vi "uTTA_Calibration.vi"() -> ()   [LabVIEW 2021]
uses:
  <vilib>/Utility/miscctls.llb/LVPointTypeDef.ctl
  uTTA_Device_Driver/CTL_uTTA_OperatingMode.ctl
  <vilib>/Analysis/6fits.llb/Curve Fitting Criteria.ctl
  <vilib>/Analysis/NI_AALBase.lvlib
  <vilib>/Analysis/NI_AALPro.lvlib
panel:
  out "Trys":i32
  out "PGA":i32
  out "Measurement Active":bool
  out "Queue":i32
  out "Communication Error":errorcluster
  out "RunTime Error":errorcluster
  out "Last Message":string
  in  "Tab Control":T1(tab)
  in  "uTTA COM":refnum<visa-resource-name>
  in  "VISA Function Gen":refnum<visa-resource-name>
  in  "Storage_Path":path=path "C:/temp/Octave_Thermal_Modelling/Measurement_Data"
  in  "VISA DMM":refnum<visa-resource-name>
  in  "Cal Adapter":bool
  in  "DAC Increments":dbl=0.025 caption="DAC Voltage\nIncrement" min=0.001 max=1.0 format="%.3p V/Step"
  in  "Start ADC Cal":bool
  out "Calibration of Channel":u32
  out "PGA setting":u32
  out "ADC Cal.":cluster{"Voltage mean":dbl, "mean":dbl}(graph)
  out "Ref. Voltage":dbl format="%#_6pV"
  out "ADC slope":dbl format="%#_4pV/Digit"
  out "ADC lin. res":dbl caption="ADC linearization\nresidue" format="%.3p"
  out "ADC intercept":dbl format="%#_6pV"
  out "PGA":u32
  out "ADC_Variance":dbl[](array[numeric]) format="%#.2g"
  out "Temp_Variance":dbl[](array[numeric]) format="%#.2g°C"
  out "Temp_Values":dbl[](array[numeric]) format="%#.1g°C"
  out "ADC_Values":dbl[](array[numeric]) format="%#.2g"
  out "Channel":u32
  in  "Complete Cal":bool
  out "Total Measurements":u32
  in  "Shunt Resistance":dbl format="%#_3pOhm"
  in  "Get Measurement":bool
  out "ADC Cal. 2":cluster{"Voltage mean":dbl, "mean":dbl}(graph)
  out "ADC_Values 2":dbl[](array[numeric]) format="%#.2g"
  out "ADC_Variance 2":dbl[](array[numeric]) format="%#.2g"
  in  "Start":bool
  out "Status":string="Exit"
  in  "stop":bool
  # "1. Connect the function generator with a 50Ohm Terminator and a BNC Y-Adaptor to the input of the uTTA.\n2. Connect a ground lead to the outer Conductor of the BNC line to provide propper grounding\n3. Start the calibration"
  # "1. Connect a power supply through a low resistance value shunt ( 10-100mOhm) to the JUT Current Input (J107) of uTTA.\n2. Connect the ground of the power supply to J106 of uTTA.\n3. Connect the sense leads of your multimeter to the sense terminals of the shunt.\n4. Set the power supply to a low current setting (~100mA).\n5. Get a measurement\n6. Set a higher current to the power supply. Steps of 1A to 2A should be sufficient.\n7. Repeat steps 5 and 6 multiple times until you have a good number of measurements.\n8. To finalize the calibration press \"Complete Calibration\"."
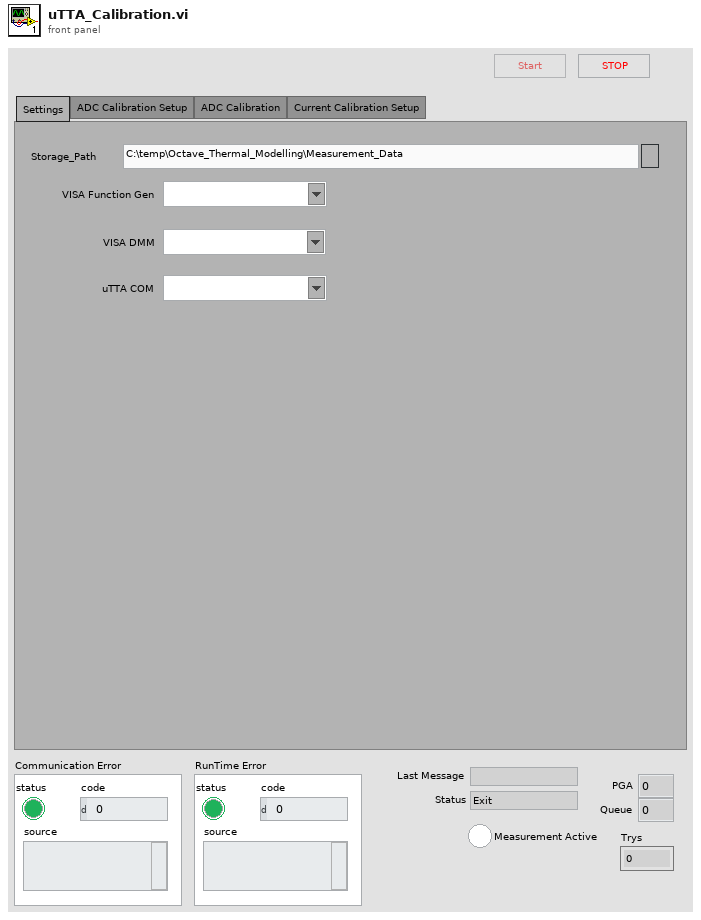
[diagram p1: front panel]
types:
  T1 = enum32{"Settings", "ADC Calibration Setup", "ADC Calibration", "Current Calibration Setup"}
  T2 = typedef "LVPointTypeDef.ctl" = cluster{"Horizontal":i16, "Vertical":i16}
  T3 = cluster{"ADC Values":i16[][], "Temperatures":dbl[][]}
  T4 = typedef "CTL_uTTA_OperatingMode.ctl" = enum16{"NORMAL", "CALIBRATION"}
  T5 = enum8{"Enabled", "Disabled", "Disabled and Grayed Out"}
  T6 = enum16{"open", "open or create", "create or replace", "create", "open (read-only)"}
  T7 = typedef "NI_AALPro.lvlib/Curve Fitting Criteria.ctl" = u16
  T8 = cluster{"CH0  CURRENT":i16[], "CH1 VOLTAGE":i16[]}
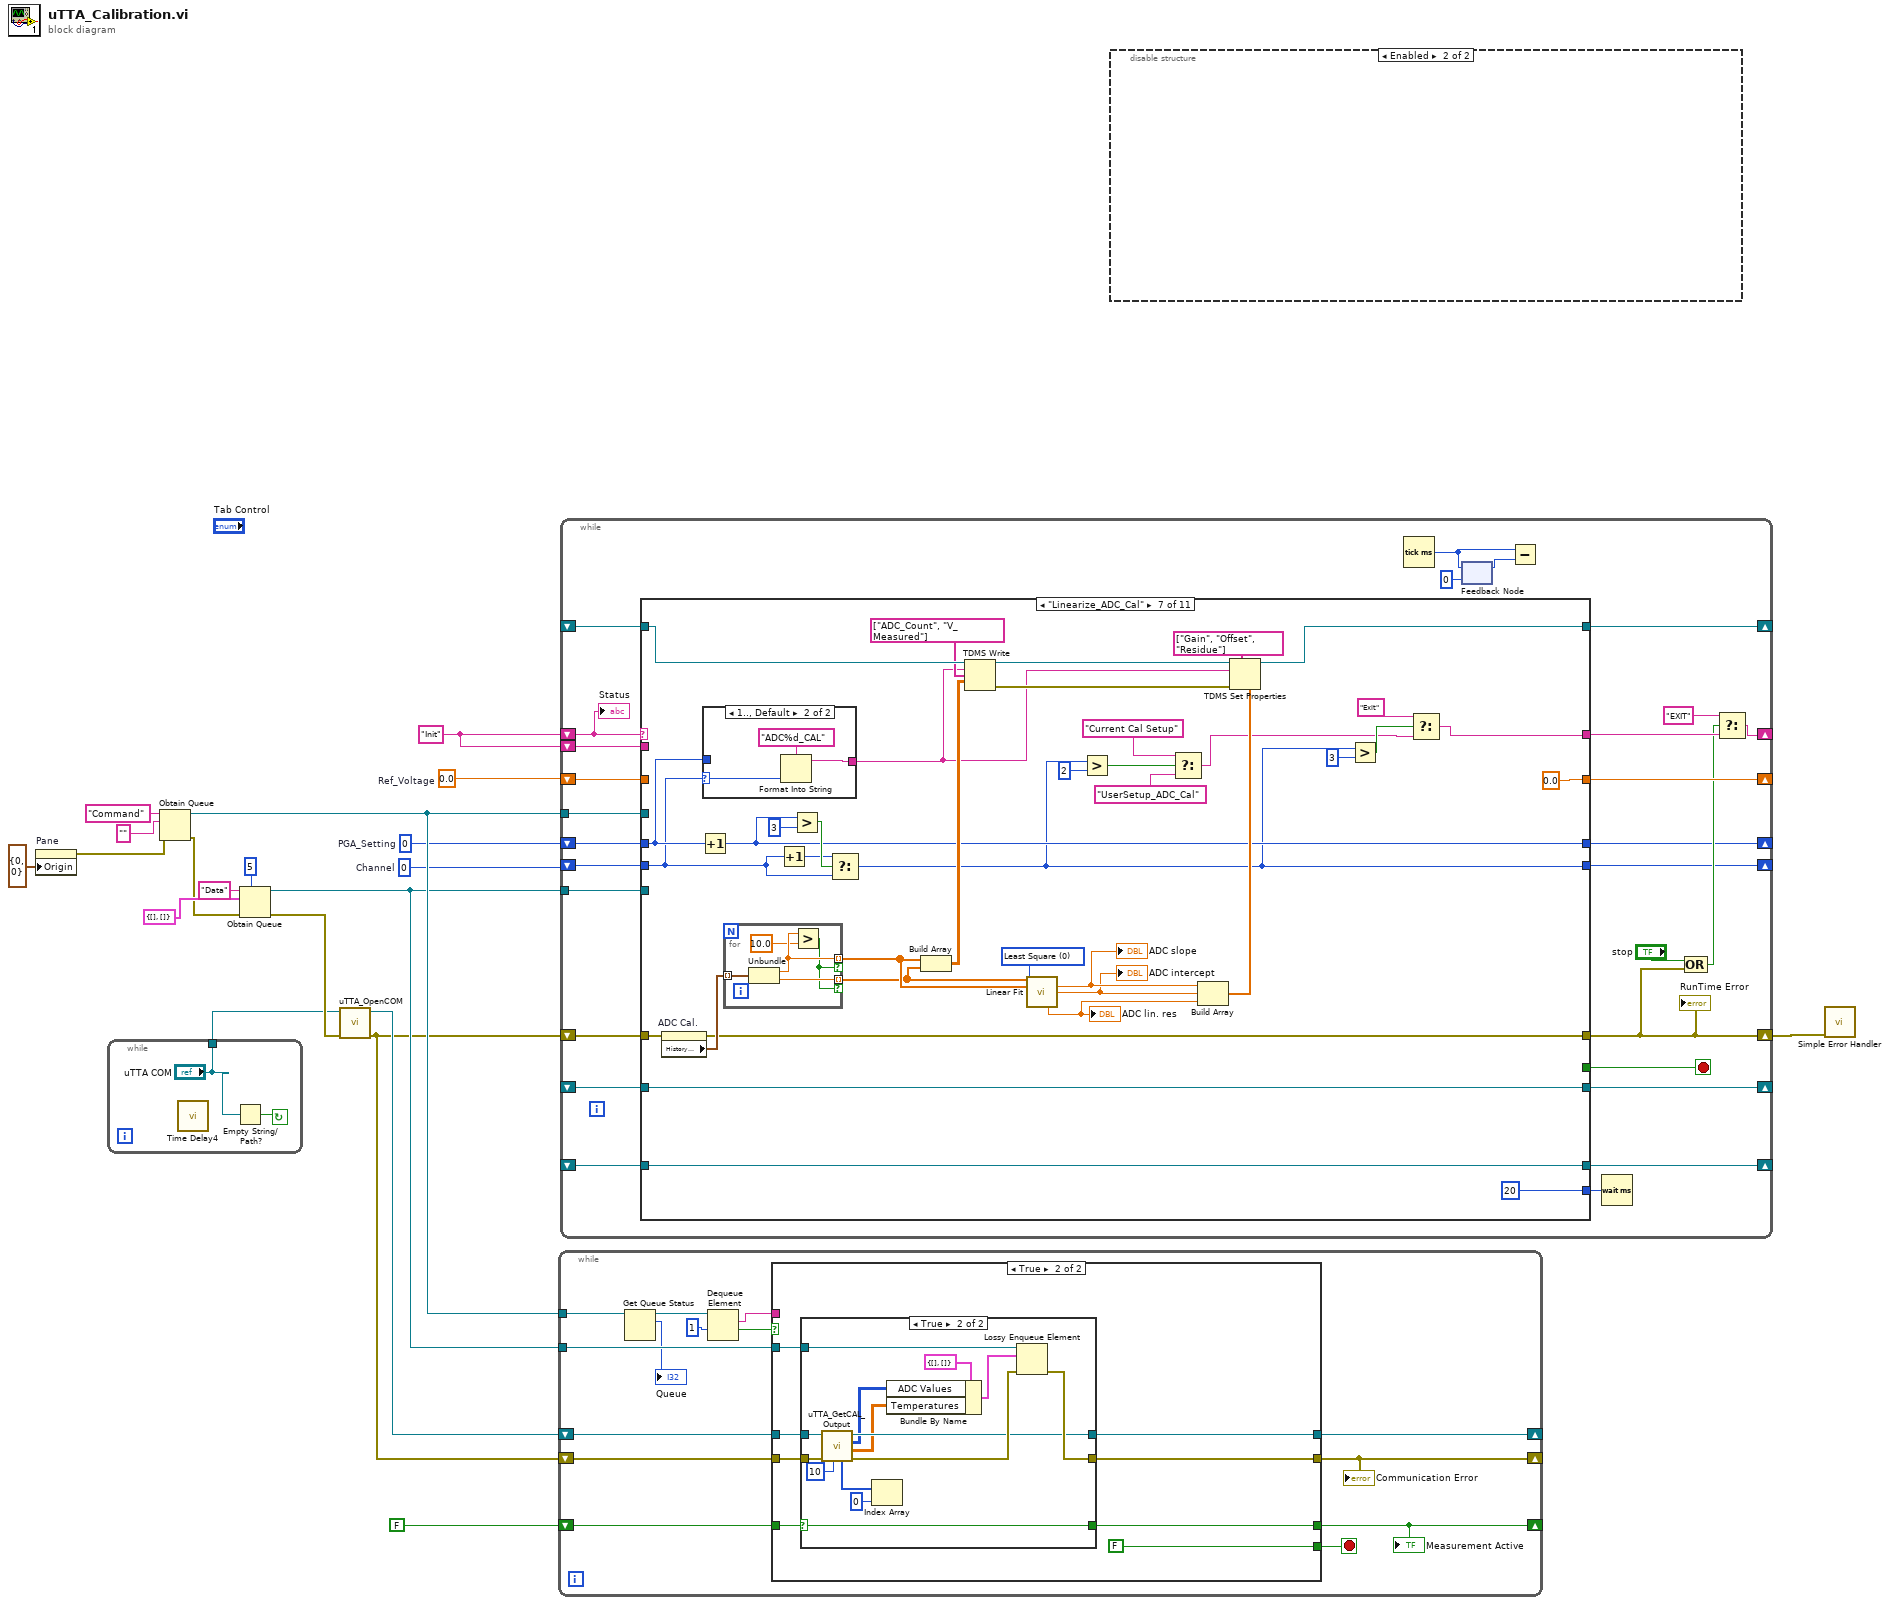
[diagram p0: block diagram]
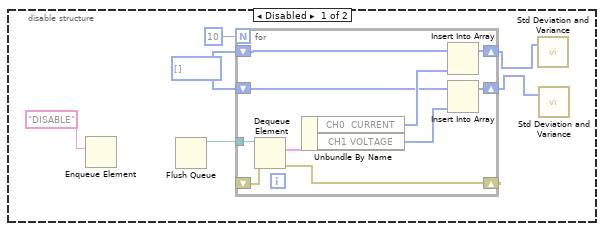
[diagram p2: hidden frame]
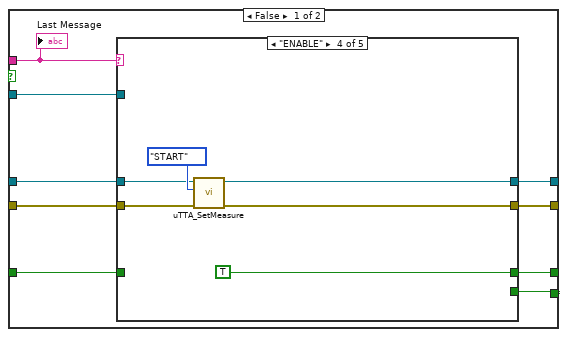
[diagram p3: hidden frame]
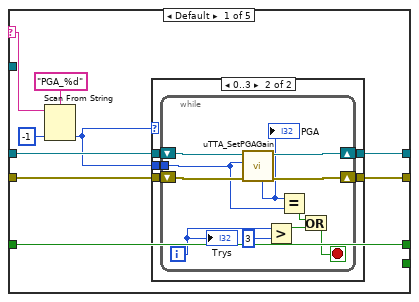
[diagram p4: hidden frame]
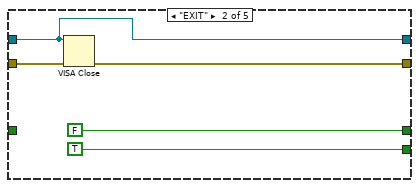
[diagram p6: hidden frame]
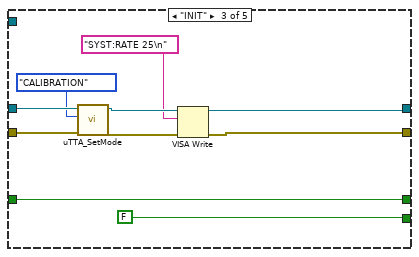
[diagram p7: hidden frame]
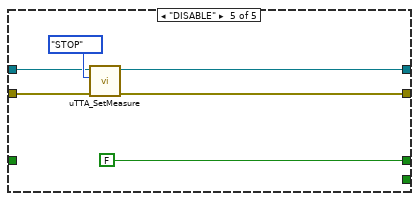
[diagram p8: hidden frame]
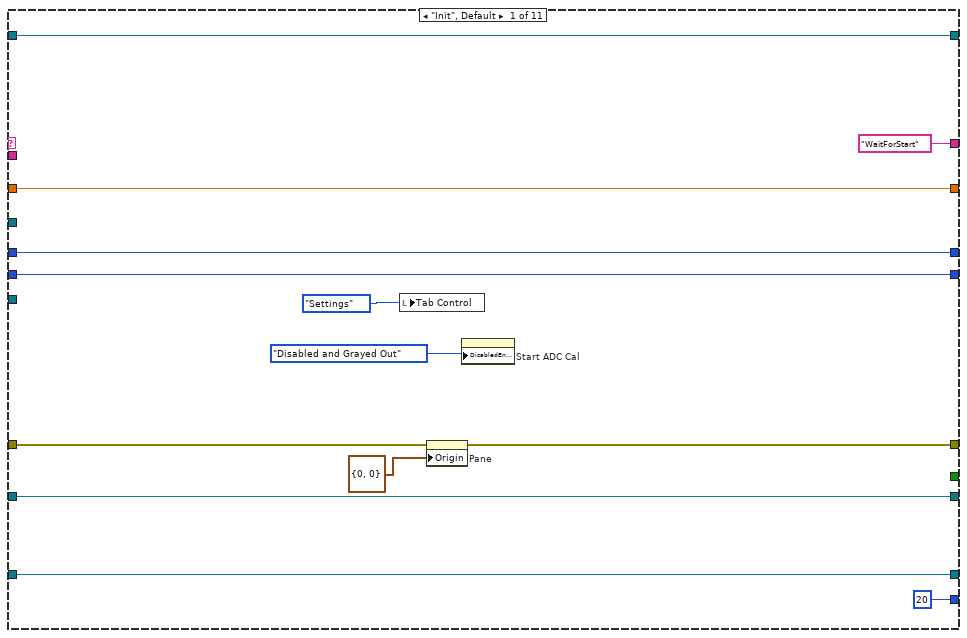
[diagram p10: hidden frame]
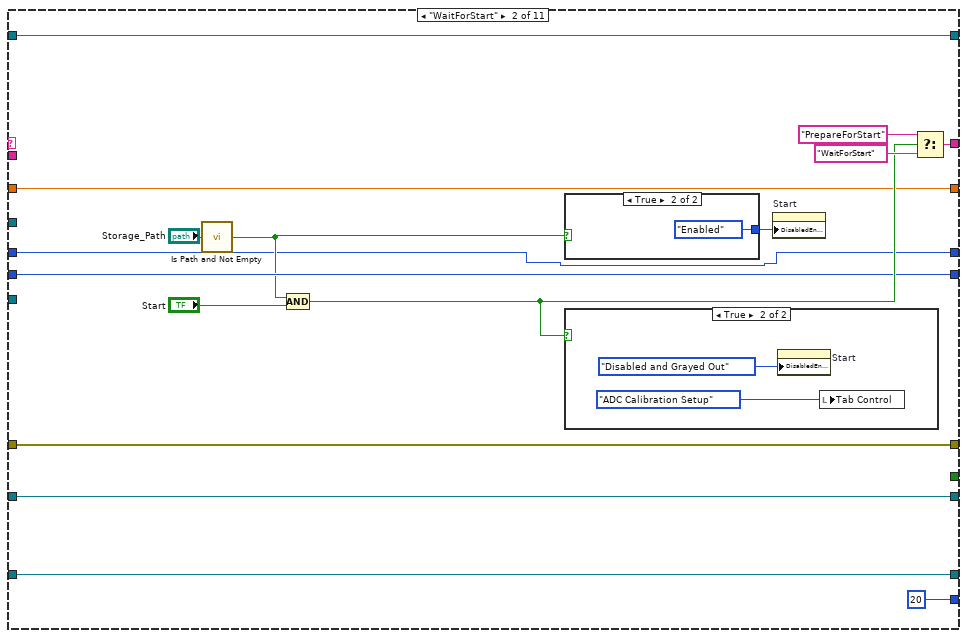
[diagram p11: hidden frame]
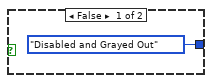
[diagram p12: hidden frame]
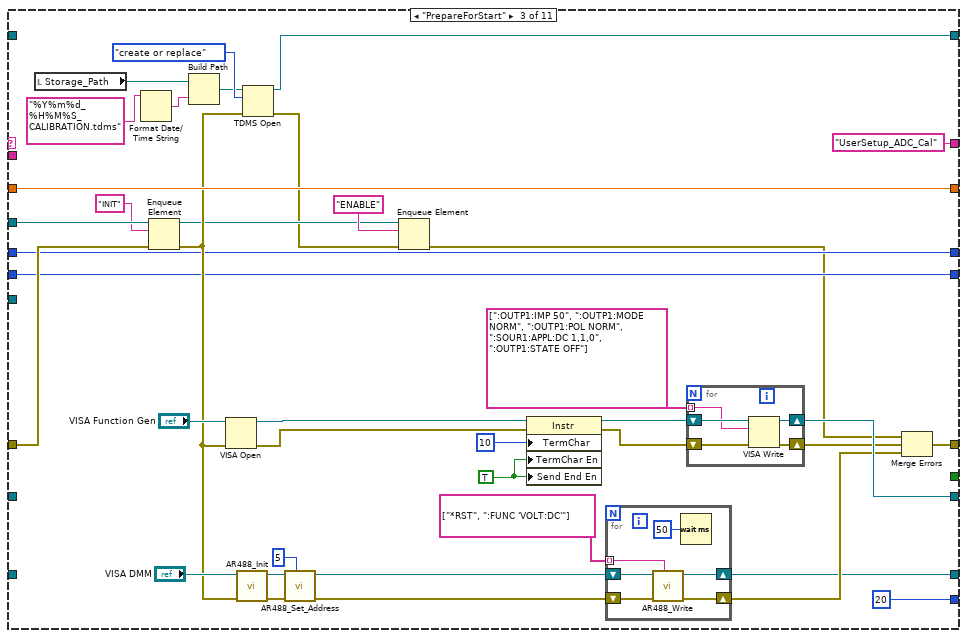
[diagram p14: hidden frame]
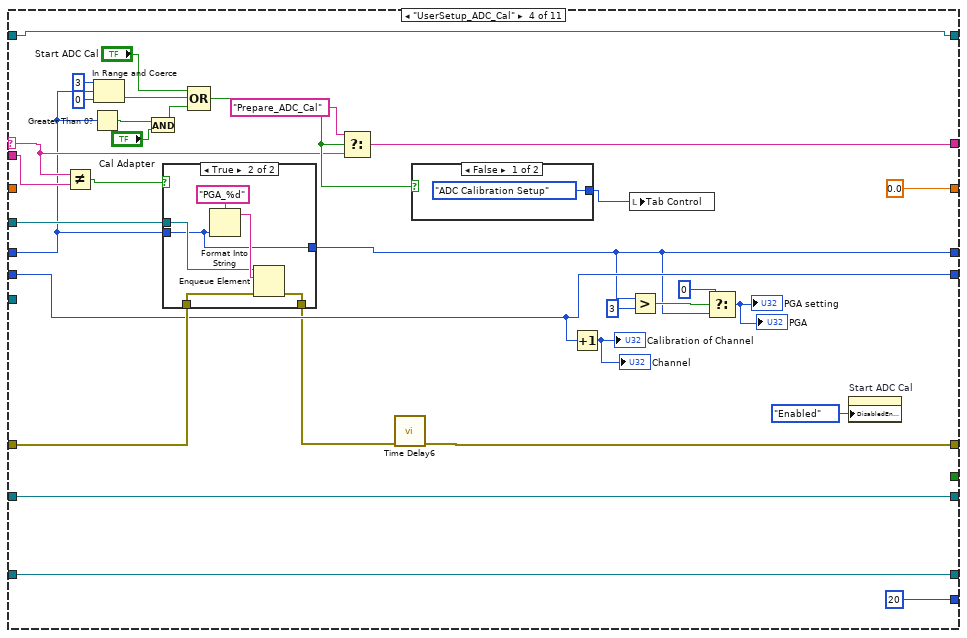
[diagram p15: hidden frame]
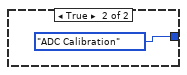
[diagram p17: hidden frame]
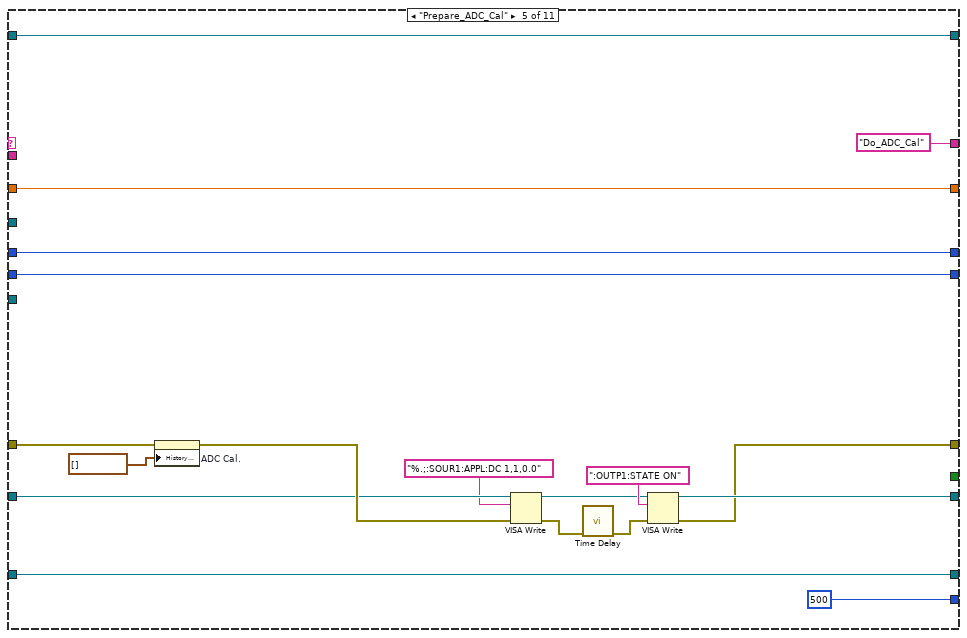
[diagram p18: hidden frame]
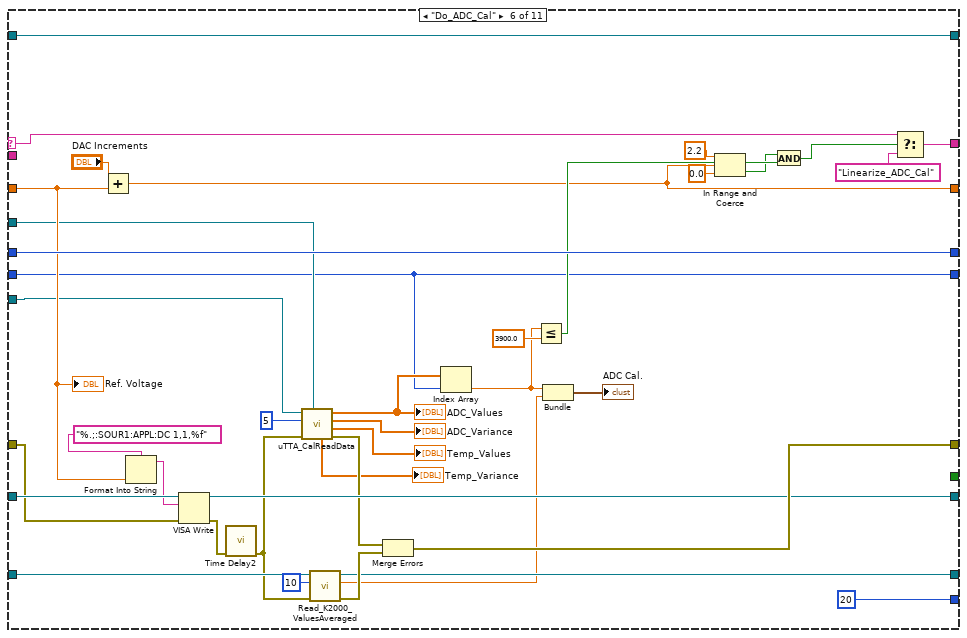
[diagram p19: hidden frame]
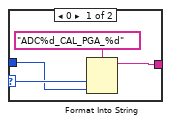
[diagram p20: hidden frame]
diagram:
  w4 = u32 0  # Channel
  w7 = u32 0  # PGA_Setting
  w11 = 0.0  # Ref_Voltage
  w10 = "Init"
  n1 = property on="Pane" class="Pane"("Origin"=T2 {"Horizontal"=0, "Vertical"=0}) -> (error out=w2:errorcluster)  [unwired: 2 in, 1 out]
  n2 = while {
    tunnel: ["uTTA COM"] -> w1
    stop <- w22 continue-if-true
    n3 = call "Time Delay4"() -> ()  [unwired: 11 in, 1 out]
    n4 = Empty String/Path?(string/path="uTTA COM") -> (empty?=w22:bool)
  }
  n5 = Obtain Queue(name (unnamed)="Command", element data type="" ("name (unnamed)"), error in (no error)=w2) -> (queue out=w14:refnum<queue>, error out=w15:errorcluster)  [unwired: 2 in, 1 out]
  n6 = Obtain Queue(max queue size (-1, unlimited)=5, name (unnamed)="Data", element data type=T3 {"ADC Values"=[], "Temperatures"=[]}, error in (no error)=w15) -> (queue out=w6:refnum<queue>, error out=w9:errorcluster)  [unwired: 1 in, 1 out]
  n7 = call "uTTA_OpenCOM.vi"("error in"=w9, "VISA in"=w1) -> ("error out"=w5:errorcluster, "VISA out"=w8:refnum<visa-resource-name>)  [unwired: 7 in, 1 out]
  n8 = while {
    shift-right: [w34] -> _
    shift-left: w8 -> [w36]
    shift-right: [w33] -> _
    shift-left: w5 -> [w35]
    tunnel: w14 -> [w30]
    tunnel: w6 -> [w31]
    shift-right: [w25] -> _
    shift-left: FALSE -> [w26]
    stop <- w32 stop-if-true
    n9 = Get Queue Status(queue=w30) -> (queue out=w24:refnum<queue>, # pending remove=→"Queue":i32)  [unwired: 2 in, 6 out]
    n10 = Dequeue Element(queue=w24, timeout in ms (-1)=1) -> (element=w27:string, timed out?=w28:bool)  [unwired: 1 in, 2 out]
    n11 = case shown="True" w28 {
      tunnel: w36 -> [w45 w105]
      tunnel: w35 -> [w44 w104]
      tunnel: [w43 w102] -> w34
      tunnel: [w42 w101] -> w33
      tunnel: [w41 FALSE] -> w32
      tunnel: w31 -> [w40 w100]
      tunnel: w27 -> [w37 _]
      tunnel: w26 -> [w39 w106]
      tunnel: [w38 w103] -> w25
      frame False {
        n12 = case shown="\"ENABLE\"" w37 {
          selector: w37 -> [w53 _ _ _ _]
          tunnel: w45 -> [w50 w73 w85 w91 w97]
          tunnel: w44 -> [w49 w75 w84 w90 w96]
          tunnel: [w48 w73 w80 w88 w95] -> w43
          tunnel: [w47 w74 w79 w89 w94] -> w42
          tunnel: [_ TRUE FALSE _ _] -> w41
          tunnel: w40 -> [_ _ _ _ _]
          tunnel: w39 -> [w54 _ w86 _ _]
          tunnel: [w54 FALSE w86 TRUE FALSE] -> w38
          frame Default {
            n13 = Scan From String(format string="PGA_%d", input string=w53, default 1=-1 ("default value 1")) -> (output 1=w46:i32)  [unwired: 2 in, 3 out]
            n14 = case shown="0..3" w46 {
              tunnel: w46 -> [_ w61]
              tunnel: w50 -> [w56 w60]
              tunnel: w49 -> [w55 w59]
              tunnel: [w56 w58] -> w48
              tunnel: [w55 w57] -> w47
              frame Default {
              }
              frame 0..3 {
                n15 = while {
                  tunnel: w61 -> [w68]
                  shift-right: [w70] -> w58
                  shift-left: w60 -> [w72]
                  shift-right: [w69] -> w57
                  shift-left: w59 -> [w71]
                  i -> [w64]
                  stop <- w67 stop-if-true
                  n16 = call "uTTA_SetPGAGain.vi"("error in"=w71, "PGA Gain"=w68, "VISA Refnum in"=w72) -> ("error out"=w69:errorcluster, "VISA Refnum out"=w70:refnum<visa-resource-name>, "Set PGA Gain"=w62:u32)  [unwired: 5 in, 1 out]
                  "PGA" <- w62
                  n17 = Greater?(x=w64, y=3) -> (0:w65:bool)
                  n18 = Equal?(x=w62, y=w68) -> (x = y?=w66:bool)
                  n19 = Or(x=w66, y=w65) -> (x .or. y?=w67:bool)
                  "Trys" <- w64
                }
              }
            }
          }
          frame "EXIT" {
            n20 = VISA Close(VISA resource name=w73, error in (no error)=w75) -> (error out=w74:errorcluster)
          }
          frame "INIT" {
            n21 = call "uTTA_SetMode.vi"("error in"=w84, "OperatingMode"=CTL_uTTA_OperatingMode."CALIBRATION", "VISA Refnum in"=w85) -> ("error out"=w81:errorcluster, "VISA Refnum out"=w82:refnum<visa-resource-name>)  [unwired: 6 in, 1 out]
            n22 = VISA Write(VISA resource name=w82, write buffer="SYST:RATE 25\n", error in (no error)=w81) -> (VISA resource name out=w80:refnum<visa-resource-name>, error out=w79:errorcluster)  [unwired: 1 out]
          }
          frame "ENABLE" {
            n23 = call "uTTA_SetMeasure.vi"("error in"=w90, "Action"=enum16{"STOP", "START"}."START", "VISA Refnum in"=w91) -> ("error out"=w89:errorcluster, "VISA Refnum out"=w88:refnum<visa-resource-name>)  [unwired: 6 in, 1 out]
          }
          frame "DISABLE" {
            n24 = call "uTTA_SetMeasure.vi"("error in"=w96, "Action"=enum16{"STOP", "START"}."STOP", "VISA Refnum in"=w97) -> ("error out"=w94:errorcluster, "VISA Refnum out"=w95:refnum<visa-resource-name>)  [unwired: 6 in, 1 out]
          }
        }
        "Last Message" <- w37
      }
      frame True {
        n25 = case shown="True" w106 {
          selector: w106 -> [w110 w124]
          tunnel: w105 -> [w109 w120]
          tunnel: w104 -> [w108 w119]
          tunnel: [w110 w124] -> w103
          tunnel: [w109 w117] -> w102
          tunnel: [w108 w121] -> w101
          tunnel: w100 -> [_ w123]
          frame False {
          }
          frame True {
            n26 = call "uTTA_GetCAL_Output.vi"("Number of Samples"=u32 10, "error in"=w119, "VISA Refnum in"=w120) -> ("error out"=w118:errorcluster, "Temperatures"=w115:dbl[][], "ADCs"=w116:i32[][], "VISA Refnum out"=w117:refnum<visa-resource-name>, "PGA"=w112:i32[])  [unwired: 4 in]
            n27 = Index Array(array=w112, index=0) -> ()  [unwired: 1 out]
            n28 = Bundle By Name(cluster=T3 {"ADC Values"=[], "Temperatures"=[]}, "ADC Values"=w116, "Temperatures"=w115) -> (w122:T3)
            n29 = Lossy Enqueue Element(queue=w123, element=w122, error in (no error)=w118) -> (error out=w121:errorcluster)  [unwired: 3 out]
          }
        }
      }
    }
    "Communication Error" <- w33
    "Measurement Active" <- w25
  }
  n30 = while {
    shift-right: [w136] -> _
    shift-left: w10 -> [w147]
    shift-right: [w134] -> w13
    shift-left: w5 -> [w152]
    shift-right: [w145] -> _
    shift-left: _ -> [w146]
    shift-right: [w144] -> _
    shift-left: _ -> [w143]
    shift-left: w10 -> [w142]
    tunnel: w14 -> [w141]
    tunnel: w6 -> [w140]
    shift-right: [w138] -> _
    shift-left: w11 -> [w139]
    shift-right: [w130] -> _
    shift-left: _ -> [w129]
    shift-right: [w127] -> _
    shift-left: w7 -> [w128]
    shift-right: [w125] -> _
    shift-left: w4 -> [w126]
    stop <- w131 stop-if-true
    n31 = case shown="\"Linearize_ADC_Cal\"" w147 {
      selector: w147 -> [_ _ _ w249 _ w329 _ _ w401 _ w477]
      tunnel: [_ _ _ _ _ _ _ _ _ _ TRUE] -> w131
      tunnel: w152 -> [w162 w181 w209 w259 w291 w319 w366 w393 w421 w431 w464]
      tunnel: ["WaitForStart" ("t") w174 "UserSetup_ADC_Cal" ("t") w267 "Do_ADC_Cal" ("t") w328 w336 "User_CurrentCal_Wait" ("t") w404 w449 w477] -> w137
      tunnel: [w158 w181 w215 w243 w287 w327 w342 w385 w421 w430 w468] -> w134
      tunnel: [u32 20 u32 20 u32 20 u32 20 u32 500 u32 20 u32 20 u32 20 u32 20 u32 20 u32 10] -> w151
      tunnel: w146 -> [w161 w173 _ w266 w282 w320 w370 w398 w420 w453 w466]
      tunnel: [w161 w173 w218 w266 w288 w318 w370 w398 w420 w453 w465] -> w145
      tunnel: [w160 w172 w194 w265 w294 w323 w368 w397 w419 w433 w470] -> w144
      tunnel: w143 -> [w160 w172 _ w265 w294 w325 w368 w397 w419 w432 w470]
      tunnel: w142 -> [_ _ _ w248 _ _ _ _ _ w449 _]
      tunnel: w141 -> [_ _ w213 w258 _ w297 _ _ _ w428 w455]
      tunnel: w140 -> [_ _ _ _ _ w306 _ _ _ w429 _]
      tunnel: w139 -> [w159 w171 w211 _ w292 w308 _ w396 w418 w452 w474]
      tunnel: [w159 w171 w211 0.0 w292 w307 0.0 w396 w418 w452 w474] -> w138
      tunnel: [w156 w169 w207 w260 w290 w321 w364 w395 w417 w451 w461] -> w130
      tunnel: w129 -> [w156 w169 _ w260 w290 w321 w365 w395 w417 w451 w461]
      tunnel: w128 -> [w153 w166 w191 w241 w286 w313 w345 w388 _ w427 w463]
      tunnel: [w153 w166 w191 w246 w286 w313 w352 w388 u32 6 ("PGA_Setting") w427 w463] -> w127
      tunnel: w126 -> [w155 w168 w190 w254 w284 w296 w343 w394 _ w450 w462]
      tunnel: [w155 w168 w190 w254 w284 w296 w340 w394 u32 3 ("Channel") w450 w462] -> w125
      frame "Init", Default {
        n32 = local write "Tab Control"(T1."Settings" ("Tab Control")) -> ()
        n33 = property on="Pane" class="Pane"(error in=w162, "Origin"=T2 {"Horizontal"=0, "Vertical"=0}) -> (error out=w158:errorcluster)  [unwired: 1 in, 1 out]
        n34 = property on="Start ADC Cal" class="Bool"("DisabledEnum"=T5."Disabled and Grayed Out" ("Disabled")) -> ()  [unwired: 2 in, 2 out]
      }
      frame "WaitForStart" {
        n35 = call <vilib>:"Is Path and Not Empty.vi"("path"="Storage_Path") -> ("Is Path and Not Empty?"=w167:bool)  [unwired: 4 in]
        n36 = Compound Arithmetic op=AND(w167, "Start") -> (w175:bool)
        n37 = case shown="True" w167 {
          tunnel: [T5."Disabled and Grayed Out" ("Disabled") T5."Enabled" ("Disabled")] -> w177
          frame False {
          }
          frame True {
          }
        }
        n38 = case shown="True" w175 {
          frame False {
          }
          frame True {
            n39 = property on="Start" class="Bool"("DisabledEnum"=T5."Disabled and Grayed Out" ("Disabled")) -> ()  [unwired: 2 in, 2 out]
            n40 = local write "Tab Control"(T1."ADC Calibration Setup" ("Tab Control")) -> ()
          }
        }
        n41 = property on="Start" class="Bool"("DisabledEnum"=w177) -> ()  [unwired: 2 in, 2 out]
        n42 = Select(t="PrepareForStart", s=w175, f="WaitForStart" ("t")) -> (s? t:f=w174:string)
      }
      frame "PrepareForStart" {
        w222 = TRUE ("Message Based Settings:Termination Character Enable")
        n43 = local read "Storage_Path"() -> (w204:path)
        n44 = Format Date/Time String(time format string (%c)="%Y%m%d_%H%M%S_CALIBRATION.tdms") -> (date/time string=w205:string)  [unwired: 2 in]
        n45 = Enqueue Element(queue=w213, element="INIT", error in (no error)=w209) -> (queue out=w188:refnum<queue>, error out=w199:errorcluster)  [unwired: 1 in, 1 out]
        n46 = Build Path(base path=w204, name or relative path=w205) -> (appended path=w203:path)
        n47 = VISA Open(error in (no error)=w199, VISA resource name="VISA Function Gen") -> (VISA resource name=w221:refnum<visa-resource-name>, error out=w220:errorcluster)  [unwired: 3 in]
        n48 = call "AR488_Init.vi"("error in (no error)"=w199, "VISA Refnum in"="VISA DMM") -> ("error out"=w197:errorcluster, "VISA Refnum out"=w198:refnum<visa-resource-name>)  [unwired: 8 in]
        n49 = TDMS Open(8:w199, 10:T6."create or replace" ("operation (0:open)"), 11:w203) -> (0:w187:errorcluster, 3:w207:refnum<k34>)  [unwired: 4 in]
        n50 = call "AR488_Set_Address.vi"("Address (0-31)"=u32 5, "error in"=w197, "VISA Refnum in"=w198) -> ("error out"=w192:errorcluster, "VISA Refnum out"=w193:refnum<visa-resource-name>)  [unwired: 7 in]
        n51 = Enqueue Element(queue=w188, element="ENABLE", error in (no error)=w187) -> (error out=w186:errorcluster)  [unwired: 1 in, 2 out]
        n52 = property class="Instr"(reference=w221, error in=w220, "TermChar"=u8 10 ("Message Based Settings:Termination Character"), "TermChar En"=w222, "Send End En"=w222) -> (reference out=w219:refnum<visa-resource-name>, error out=w217:errorcluster)
        n53 = for {
          tunnel: string[] ["*RST", ":FUNC 'VOLT:DC'"] -> [w229] mode=indexing
          shift-right: [w227] -> w194
          shift-left: w193 -> [w230]
          shift-right: [w226] -> w195
          shift-left: w192 -> [w228]
          n54 = call "AR488_Write.vi"("write"=w229, "error in (no error)"=w228, "VISA Refnum in"=w230) -> ("error out"=w226:errorcluster, "VISA Refnum out"=w227:refnum<visa-resource-name>)  [unwired: 7 in]
          n55 = Wait (ms)(milliseconds to wait=u32 50) -> ()  [unwired: 1 out]
        }
        n56 = for {
          shift-right: [w234] -> w218
          shift-left: w219 -> [w235]
          tunnel: string[] [":OUTP1:IMP 50", ":OUTP1:MODE NORM", ":OUTP1:POL NORM", ":SOUR1:APPL:DC 1,1,0", ":OUTP1:STATE OFF"] ("Array 2") -> [w233] mode=indexing
          shift-right: [w231] -> w216
          shift-left: w217 -> [w232]
          n57 = VISA Write(VISA resource name=w235, write buffer=w233, error in (no error)=w232) -> (VISA resource name out=w234:refnum<visa-resource-name>, error out=w231:errorcluster)  [unwired: 1 out]
        }
        n58 = Merge Errors(w186, w216, w195) -> (w215:errorcluster)
      }
      frame "UserSetup_ADC_Cal" {
        n59 = Not Equal?(x=w249, y=w248) -> (x != y?=w247:bool)
        n60 = Greater Than 0?(x=w241) -> (x > 0?=w239:bool)
        n61 = In Range and Coerce(upper limit=u32 3, x=w241, lower limit=u32 0) -> (In Range?=w250:bool)  [unwired: 1 out]
        n62 = And(x=w239, y="Cal Adapter") -> (x .and. y?=w238:bool)
        n63 = case shown="True" w247 {
          tunnel: w259 -> [w269 w275]
          tunnel: [w269 w274] -> w244
          tunnel: w258 -> [_ w271]
          tunnel: w241 -> [w268 w270]
          tunnel: [w268 w270] -> w246
          frame False {
          }
          frame True {
            n64 = Format Into String(format string="PGA_%d" ("element"), w270) -> (resulting string=w272:string)  [unwired: 2 in, 1 out]
            n65 = Enqueue Element(queue=w271, element=w272, error in (no error)=w275) -> (error out=w274:errorcluster)  [unwired: 1 in, 2 out]
          }
        }
        n66 = Compound Arithmetic op=OR("Start ADC Cal", w250, w238) -> (w252:bool)
        n67 = Select(t="Prepare_ADC_Cal", s=w252, f=w249) -> (s? t:f=w267:string)
        n68 = call "Time Delay6"("error in (no error)"=w244) -> ("error out"=w243:errorcluster)  [unwired: 10 in]
        n69 = case shown="False" w252 {
          tunnel: [T1."ADC Calibration Setup" ("Tab Control") T1."ADC Calibration" ("Tab Control")] -> w245
          frame False {
          }
          frame True {
          }
        }
        n70 = Increment(x=w254) -> (x+1=→"Calibration of Channel" →"Channel":u32)
        n71 = local write "Tab Control"(w245) -> ()
        n72 = Greater?(x=w246, y=u32 3) -> (0:w256:bool)
        n73 = Select(t=u32 0, s=w256, f=w246) -> (s? t:f=→"PGA" →"PGA setting":u32)
        n74 = property on="Start ADC Cal" class="Bool"("DisabledEnum"=T5."Enabled" ("Disabled")) -> ()  [unwired: 2 in, 2 out]
      }
      frame "Prepare_ADC_Cal" {
        n75 = property on="ADC Cal." class="WFChart (strict)"(error in=w291, "History Data"=cluster{"Voltage mean":dbl, "mean":dbl}[] []) -> (error out=w283:errorcluster)  [unwired: 1 in, 1 out]
        n76 = VISA Write(VISA resource name=w282, write buffer="%.;:SOUR1:APPL:DC 1,1,0.0", error in (no error)=w283) -> (VISA resource name out=w280:refnum<visa-resource-name>, error out=w279:errorcluster)  [unwired: 1 out]
        n77 = call "Time Delay"("error in (no error)"=w279) -> ("error out"=w278:errorcluster)  [unwired: 10 in]
        n78 = VISA Write(VISA resource name=w280, write buffer=":OUTP1:STATE ON", error in (no error)=w278) -> (VISA resource name out=w288:refnum<visa-resource-name>, error out=w287:errorcluster)  [unwired: 1 out]
      }
      frame "Do_ADC_Cal" {
        n79 = Add(x="DAC Increments", y=w308) -> (x+y=w307:dbl)
        n80 = Format Into String(format string="%.;:SOUR1:APPL:DC 1,1,%f" ("write buffer"), w308) -> (resulting string=w315:string)  [unwired: 2 in, 1 out]
        n81 = VISA Write(VISA resource name=w320, write buffer=w315, error in (no error)=w319) -> (VISA resource name out=w318:refnum<visa-resource-name>, error out=w317:errorcluster)  [unwired: 1 out]
        n82 = call "Time Delay2"("error in (no error)"=w317) -> ("error out"=w305:errorcluster)  [unwired: 10 in]
        n83 = call "uTTA_CalReadData.vi"("Control Queue"=w297, "error in"=w305, "Averaged Values"=5, "Data Queue in"=w306) -> ("error out"=w304:errorcluster, "Temp_Values"=→"Temp_Values":dbl[], "ADC_Variance"=→"ADC_Variance":dbl[], "ADC_Values"=w299:dbl[], "Temp_Variance"=→"Temp_Variance":dbl[])  [unwired: 3 in]
        "ADC_Values" <- w299
        n84 = call "Read_K2000_ValuesAveraged.vi"("error in"=w305, "No. Averaged Values"=10, "VISA Refnum in"=w325) -> ("error out"=w324:errorcluster, "mean"=w314:dbl, "VISA Refnum out"=w323:refnum<visa-resource-name>)  [unwired: 6 in]
        n85 = Merge Errors(w304, w324) -> (w327:errorcluster)
        n86 = Index Array(array=w299, index=w296) -> (element=w298:dbl)
        n87 = Less Or Equal?(x=w298, y=3900.0) -> (x <= y?=w311:bool)
        n88 = Bundle("mean"=w298, "mean"=w314) -> (→"ADC Cal.":cluster{"mean":dbl, "mean":dbl})  [unwired: 1 in]
        n89 = In Range and Coerce(upper limit=2.2, x=w307, lower limit=0.0) -> (In Range?=w310:bool)  [unwired: 1 out]
        n90 = And(x=w310, y=w311) -> (x .and. y?=w309:bool)
        n91 = Select(t=w329, s=w309, f="Linearize_ADC_Cal") -> (s? t:f=w328:string)
        "Ref. Voltage" <- w308
      }
      frame "Linearize_ADC_Cal" {
        w371 = T7 0 items=["Least Square", "Least Absolute Residual", "Bisquare"] ("method")
        n92 = property on="ADC Cal." class="WFChart (strict)"(error in=w366) -> (error out=w342:errorcluster, "History Data"=w372:cluster{"Voltage mean":dbl, "mean":dbl}[])  [unwired: 1 in, 1 out]
        n93 = Increment(x=w345) -> (x+1=w352:u32)
        n94 = case shown="1.., Default" w343 {
          selector: w343 -> [w374 w377]
          tunnel: w345 -> [w373 _]
          tunnel: [w375 w378] -> w344
          frame 0 {
            n95 = Format Into String(format string="ADC%d_CAL_PGA_%d" ("group name in (Untitled)"), w374, w373) -> (resulting string=w375:string)  [unwired: 2 in, 1 out]
          }
          frame 1.., Default {
            n96 = Format Into String(format string="ADC%d_CAL" ("group name in (Untitled)"), w377) -> (resulting string=w378:string)  [unwired: 2 in, 1 out]
          }
        }
        n97 = for {
          tunnel: w372 -> [w384] mode=indexing
          tunnel: [w383] -> w356 mode=indexing if=w380
          tunnel: [w382] -> w357 mode=indexing if=w380
          n98 = Unbundle(w384) -> ("Voltage mean"=w382:dbl, "mean"=w383:dbl)
          n99 = Greater?(x=w382, y=10.0) -> (0:w380:bool)
        }
        n100 = Increment(x=w343) -> (x+1=w353:u32)
        n101 = Greater?(x=w352, y=u32 3) -> (0:w354:bool)
        n102 = Select(t=w353, s=w354, f=w343) -> (s? t:f=w340:u32)
        n103 = Build Array(w357, w356) -> (w363:dbl[][])
        n104 = TDMS Write(0:w365, 5:w344, 7:string[] ["ADC_Count", "V_Measured"], 9:w363) -> (4:w348:refnum<k34>, 15:w347:errorcluster)  [unwired: 2 in, 2 out]
        n105 = call <vilib>:"Linear Fit.vi"("Y"=w356, "X"=w357, "method"=w371) -> ("slope"=w362:dbl, "intercept"=w361:dbl, "residue"=w341:dbl)  [unwired: 8 in, 2 out]
        "ADC intercept" <- w361
        "ADC lin. res" <- w341
        "ADC slope" <- w362
        n106 = Greater?(x=w340, y=u32 2) -> (0:w350:bool)
        n107 = Select(t="Current Cal Setup", s=w350, f="UserSetup_ADC_Cal" ("t")) -> (s? t:f=w337:string)
        n108 = Build Array(w362, w361, w341) -> (w360:dbl[])
        n109 = TDMS Set Properties(5:w360, 7:string[] ["Gain", "Offset", "Residue"] ("property names"), 8:w347, 10:w344, 11:w348) -> (3:w364:refnum<k34>)  [unwired: 1 in, 3 out]
        n110 = Greater?(x=w340, y=u32 3) -> (0:w338:bool)
        n111 = Select(t="Exit", s=w338, f=w337) -> (s? t:f=w336:string)
      }
      frame "Current Cal Setup" {
        w387 = cluster{"Voltage mean":dbl, "mean":dbl}[] [] ("History Data")
        n112 = property on="ADC Cal." class="WFChart (strict)"(error in=w393, "History Data"=w387) -> (error out=w386:errorcluster)  [unwired: 1 in, 1 out]
        n113 = property on="ADC Cal. 2" class="WFChart (strict)"(error in=w386, "History Data"=w387) -> (error out=w385:errorcluster)  [unwired: 1 in, 1 out]
        n114 = local write "Tab Control"(T1."Current Calibration Setup" ("Tab Control")) -> ()
        "Total Measurements" <- u32 0 ("Total Measurements")
      }
      frame "User_CurrentCal_Wait" {
        n115 = local read "Total Measurements"() -> (w413:u32)
        n116 = Greater Than 0?(x="Shunt Resistance") -> (x > 0?=w412:bool)
        n117 = Greater?(x=w413, y=u32 6) -> (0:w414:bool)
        n118 = And(x="Get Measurement", y=w412) -> (x .and. y?=w411:bool)
        n119 = case shown="False" w412 {
          tunnel: [T5."Disabled and Grayed Out" ("Disabled") T5."Enabled" ("Disabled")] -> w403
          frame False {
          }
          frame True {
          }
        }
        n120 = case shown="False" w414 {
          tunnel: [T5."Disabled and Grayed Out" ("Disabled") T5."Enabled" ("Disabled")] -> w402
          frame False {
          }
          frame True {
          }
        }
        n121 = Select(t="Do_Measurement", s=w411, f=w401) -> (s? t:f=w415:string)
        n122 = property on="Get Measurement" class="Bool"("DisabledEnum"=w403) -> ()  [unwired: 2 in, 2 out]
        n123 = property on="Complete Cal" class="Bool"("DisabledEnum"=w402) -> ()  [unwired: 2 in, 2 out]
        n124 = Select(t="Linearize_ADC_Cal", s="Complete Cal", f=w415) -> (s? t:f=w404:string)
      }
      frame "Do_Measurement" {
        n125 = call "Time Delay5"("error in (no error)"=w431) -> ("error out"=w439:errorcluster)  [unwired: 10 in]
        n126 = local read "Total Measurements"() -> (w447:u32)
        n127 = call "uTTA_CalReadData.vi"("Control Queue"=w428, "error in"=w439, "Averaged Values"=5, "Data Queue in"=w429) -> ("error out"=w440:errorcluster, "ADC_Variance"=→"ADC_Variance 2":dbl[], "ADC_Values"=w442:dbl[])  [unwired: 3 in, 2 out]
        "ADC_Values 2" <- w442
        n128 = call "Read_K2000_ValuesAveraged.vi"("error in"=w439, "No. Averaged Values"=10, "VISA Refnum in"=w432) -> ("error out"=w438:errorcluster, "mean"=w445:dbl, "VISA Refnum out"=w433:refnum<visa-resource-name>)  [unwired: 6 in]
        n129 = Merge Errors(w440, w438) -> (w430:errorcluster)
        n130 = local read "Shunt Resistance"() -> (w444:dbl)
        n131 = Increment(x=w447) -> (x+1=w448:u32)
        n132 = Index Array(array=w442, index=3) -> (element=w443:dbl)
        n133 = local write "Total Measurements"(w448) -> ()
        n134 = Divide(x=w445, y=w444) -> (x/y=w446:dbl)
        n135 = Bundle("mean"=w443, w446) -> (w426:cluster{"mean":dbl, dbl})  [unwired: 1 in]
        "ADC Cal. 2" <- w426
        n136 = local write "ADC Cal."(w426) -> ()
      }
      frame "Exit" {
        n137 = Enqueue Element(queue=w455, element="DISABLE") -> (queue out=w456:refnum<queue>)  [unwired: 2 in, 2 out]
        n138 = for {
          shift-right: [w481] -> w465
          shift-left: w466 -> [w482]
          tunnel: string[] [":OUTP1:IMP 50", ":OUTP1:MODE NORM", ":OUTP1:POL NORM", ":SOUR1:APPL:DC 1,1,0", ":OUTP1:STATE OFF"] ("Array 2") -> [w480] mode=indexing
          shift-right: [w478] -> w460
          shift-left: w464 -> [w479]
          n139 = VISA Write(VISA resource name=w482, write buffer=w480, error in (no error)=w479) -> (VISA resource name out=w481:refnum<visa-resource-name>, error out=w478:errorcluster)  [unwired: 1 out]
        }
        n140 = TDMS Close(8:w460, 11:w461) -> (0:w458:errorcluster)  [unwired: 1 out]
        n141 = Flush Queue(queue=w456, error in (no error)=w458) -> (queue out=w459:refnum<queue>, error out=w457:errorcluster)  [unwired: 1 out]
        n142 = call "Time Delay3"("error in (no error)"=w457) -> ("error out"=w472:errorcluster)  [unwired: 10 in]
        n143 = Enqueue Element(queue=w459, element="EXIT", error in (no error)=w472) -> (error out=w469:errorcluster)  [unwired: 1 in, 2 out]
        n144 = VISA Close(VISA resource name=w465, error in (no error)=w469) -> (error out=w471:errorcluster)
        n145 = VISA Close(VISA resource name=w470, error in (no error)=w471) -> (error out=w468:errorcluster)
      }
    }
    "RunTime Error" <- w134
    n146 = Tick Count (ms)() -> (millisecond timer value=w149:u32)
    n147 = feedback #1(u32 0 ("millisecond timer value")) -> (w150:u32)
    n148 = feedback-in #1(w149) -> ()
    n149 = Subtract(x=w149, y=w150) -> ()  [unwired: 1 out]
    n150 = Wait (ms)(milliseconds to wait=w151) -> ()  [unwired: 1 out]
    n151 = Compound Arithmetic op=OR("stop", w134) -> (w133:bool)
    n152 = Select(t="EXIT", s=w133, f=w137) -> (s? t:f=w136:string)
    "Status" <- w147
  }
  n153 = disable-structure shown="Enabled" {
    frame Disabled {
      w485 = i16[] []
      n154 = Enqueue Element(element="DISABLE") -> ()  [unwired: 3 in, 3 out]
      n155 = Flush Queue() -> (queue out=w483:refnum<queue>)  [unwired: 2 in, 2 out]
      n156 = for {
        N: 10 -> [_]
        tunnel: w483 -> [w498]
        shift-right: [w495] -> _
        shift-left: _ -> [w497]
        shift-right: [w492] -> w486
        shift-left: w485 -> [w490]
        shift-right: [w491] -> w487
        shift-left: w485 -> [w489]
        n157 = Dequeue Element(queue=w498, error in (no error)=w497) -> (element=w496:T8, error out=w495:errorcluster)  [unwired: 1 in, 2 out]
        n158 = Unbundle By Name(w496) -> ("CH0  CURRENT"=w494:i16[], "CH1 VOLTAGE"=w493:i16[])
        n159 = Insert Into Array(array=w490, new element=w494) -> (w492:i16[])  [unwired: 1 in]
        n160 = Insert Into Array(array=w489, new element=w493) -> (w491:i16[])  [unwired: 1 in]
      }
      n161 = call <vilib>:"Std Deviation and Variance.vi"("X"=w486) -> ()  [unwired: 1 in, 3 out]
      n162 = call <vilib>:"Std Deviation and Variance.vi"("X"=w487) -> ()  [unwired: 1 in, 3 out]
    }
    frame Enabled {
    }
  }
  n163 = call <vilib>:"Simple Error Handler.vi"("error in (no error)"=w13) -> ()  [unwired: 4 in, 5 out]
